vi "calculate the percentage.vi"(11 "run statistics in":T1) -> (3 "run statistics out":T1)   [LabVIEW 2024]
uses:
  CTRLS/run statistics.ctl
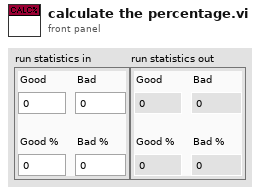
[diagram p1: front panel]
types:
  T1 = typedef "run statistics.ctl" = cluster{"Good":dbl, "Bad":dbl, "Good %":dbl, "Bad %":dbl}
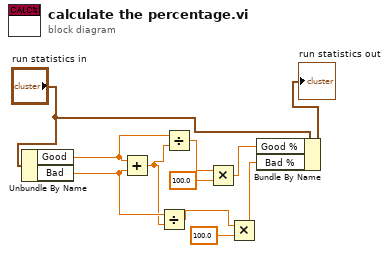
[diagram p0: block diagram]
diagram:
  n1 = Unbundle By Name("run statistics in") -> ("Good"=w11:dbl, "Bad"=w8:dbl)
  n2 = Add(x=w11, y=w8) -> (x+y=w7:dbl)
  n3 = Divide(x=w8, y=w7) -> (x/y=w5:dbl)
  n4 = Divide(x=w11, y=w7) -> (x/y=w10:dbl)
  n5 = Multiply(x=w10, y=100.0) -> (x*y=w4:dbl)
  n6 = Multiply(x=w5, y=100.0) -> (x*y=w3:dbl)
  n7 = Bundle By Name(cluster="run statistics in", "Good %"=w4, "Bad %"=w3) -> (→"run statistics out":T1)
